vi "Setup Check (SubVI).vi"(6 "[error source] (\" \")":string, 7 "Labels Array":string[](array[string]), 8 "error in (no error)":errorcluster, 9 "[error source] (\" \") 2":string, 10 "Boolean Array":bool[](array[boolean]), 11 "Channel Array":tag[](array[tag])) -> (0 "error out":errorcluster, 3 "Cluster Array Out":T1(array[cluster]))   [LabVIEW 2011]
uses:
  <vilib>/Utility/error.llb/DialogType.ctl
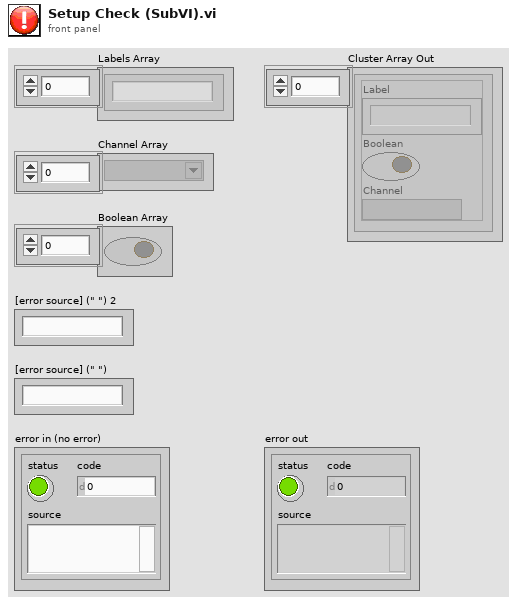
[diagram p1: front panel]
types:
  T1 = cluster{"Label":string, "Boolean":bool, "Channel":tag}[]
  T2 = typedef "DialogType.ctl" = u16
  T3 = cluster{"Label":string, "Boolean":bool, "Channel":tag}
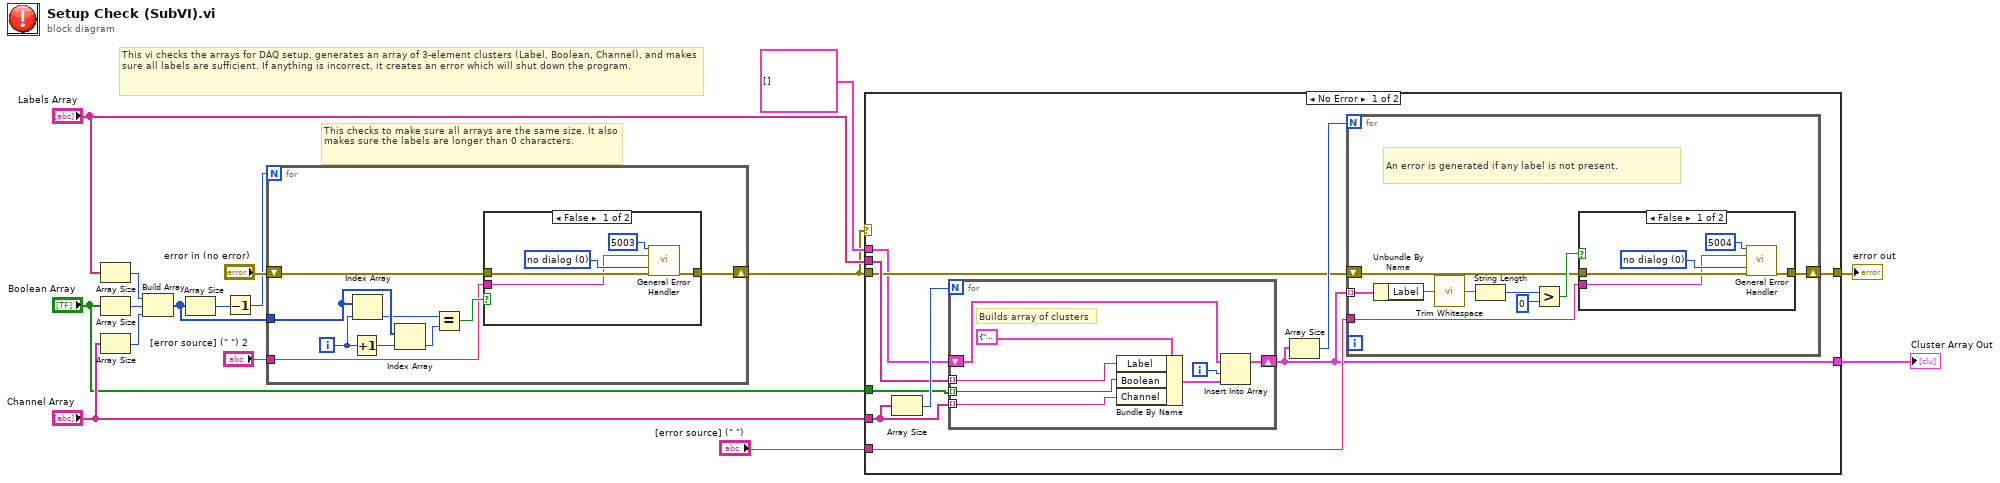
[diagram p0: block diagram]
diagram:
  # "This vi checks the arrays for DAQ setup, generates an array of 3-element clusters (Label, Boolean, Channel), and makes sure all labels are sufficient. If anything is incorrect, it creates an error which will shut down the program."
  # "This checks to make sure all arrays are the same size. It also makes sure the labels are longer than 0 characters."
  n1 = Array Size(array="Labels Array") -> (size(s)=w1:i32)
  n2 = Array Size(array="Boolean Array") -> (size(s)=w2:i32)
  n3 = Array Size(array="Channel Array") -> (size(s)=w3:i32)
  n4 = Build Array(w1, w2, w3) -> (w7:i32[])
  n5 = Array Size(array=w7) -> (size(s)=w4:i32)
  n6 = Decrement(x=w4) -> (x-1=w5:i32)
  n7 = for {
    N: w5 -> [_]
    tunnel: w7 -> [w25]
    tunnel: "[error source] (\" \") 2" -> [w17]
    shift-right: [w18] -> w9
    shift-left: "error in (no error)" -> [w19]
    i -> [w23]
    n8 = Increment(x=w23) -> (x+1=w24:i32)
    n9 = Index Array(array=w25, index=w23) -> (element=w22:i32)
    n10 = Index Array(array=w25, index=w24) -> (element=w21:i32)
    n11 = Equal?(x=w22, y=w21) -> (x = y?=w20:bool)
    n12 = case shown="False" w20 {
      tunnel: w19 -> [w30 w31]
      tunnel: [w29 w31] -> w18
      tunnel: w17 -> [w26 _]
      frame False {
        w28 = T2 0 items=["no dialog", "OK message", "continue or stop message", "OK message + warnings", "continue/stop + warnings"] ("type of dialog (OK msg:1)")
        n13 = call <vilib>:"General Error Handler.vi"("[error code] (0)"=5003, "[error source] (\" \")"=w26, "type of dialog (OK msg:1)"=w28, "error in (no error)"=w30) -> ("error out"=w29:errorcluster)  [unwired: 7 in, 4 out]
      }
      frame True {
      }
    }
  }
  n14 = case shown="No Error" w9 {
    tunnel: "Labels Array" -> [w39 _]
    tunnel: "Boolean Array" -> [w38 _]
    tunnel: "Channel Array" -> [w40 _]
    tunnel: [w34 w66] -> w11
    tunnel: w9 -> [w35 w66]
    tunnel: "[error source] (\" \")" -> [w36 _]
    tunnel: T1 [] -> [w33 w65]
    tunnel: [w32 w65] -> w16
    frame No Error {
      n15 = Array Size(array=w40) -> (size(s)=w41:i32)
      n16 = for {
        N: w41 -> [_]
        tunnel: w38 -> [w63] mode=indexing
        tunnel: w40 -> [w64] mode=indexing
        tunnel: w39 -> [w62] mode=indexing
        shift-right: [w60] -> w32
        shift-left: w33 -> [w59]
        i -> [w58]
        # "Builds array of clusters"
        n17 = Bundle By Name(cluster=T3 {"Label"="", "Boolean"=TRUE, "Channel"=""}, "Label"=w62, "Boolean"=w63, "Channel"=w64) -> (w61:T3)
        n18 = Insert Into Array(array=w59, index=w58, new element=w61) -> (w60:T1)
      }
      n19 = Array Size(array=w32) -> (size(s)=w37:i32)
      n20 = for {
        N: w37 -> [_]
        tunnel: w32 -> [w50] mode=indexing
        shift-right: [w43] -> w34
        shift-left: w35 -> [w44]
        tunnel: w36 -> [w42]
        # "An error is generated if any label is not present."
        n21 = Unbundle By Name(w50) -> ("Label"=w49:string)
        n22 = call <vilib>:"Trim Whitespace.vi"("string"=w49) -> ("trimmed string"=w48:string)  [unwired: 1 in]
        n23 = String Length(string=w48) -> (length=w47:i32)
        n24 = Greater?(x=w47, y=0) -> (0:w45:bool)
        n25 = case shown="False" w45 {
          tunnel: w44 -> [w53 w56]
          tunnel: [w52 w56] -> w43
          tunnel: w42 -> [w51 _]
          frame False {
            w54 = T2 0 items=["no dialog", "OK message", "continue or stop message", "OK message + warnings", "continue/stop + warnings"] ("type of dialog (OK msg:1)")
            n26 = call <vilib>:"General Error Handler.vi"("[error code] (0)"=5004, "[error source] (\" \")"=w51, "type of dialog (OK msg:1)"=w54, "error in (no error)"=w53) -> ("error out"=w52:errorcluster)  [unwired: 7 in, 4 out]
          }
          frame True {
          }
        }
      }
    }
    frame Error {
    }
  }
  "Cluster Array Out" <- w16
  "error out" <- w11
